vi "Set Log Trigger Default Value.vi"(8 "error in":errorcluster, 10 "log trigger default value":bool, 11 "log file in":T1 format="%.0x") -> (0 "error out":errorcluster, 3 "log file out":T1 format="%.0x")   [LabVIEW 2027, in "Embedded Data Logger Scripting.lvlib"]
uses:
  Embedded Data Logger Scripting.lvlib
  <vilib>/NI VeriStand/Custom Device API/Custom Device Item Ref.ctl
  Shared/Constants.vi
  <vilib>/NI VeriStand/Custom Device Tools/Custom Device Utility Library/NI VeriStand - Search for Item by GUID.vi
  <vilib>/NI VeriStand/Custom Device Tools/Custom Device Utility Library/Custom Device Utility Library.lvlib
  Shared/Embedded Data Logger Shared.lvlib
  <vilib>/NI VeriStand/Custom Device API/Custom Device API.lvlib
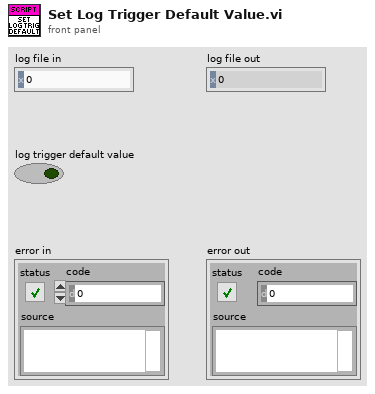
[diagram p1: front panel]
types:
  T1 = typedef "Custom Device API.lvlib/Custom Device Item Ref.ctl" = u64
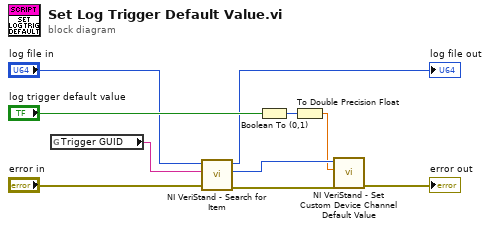
[diagram p0: block diagram]
diagram:
  n1 = global read "Constants.vi" "Trigger GUID"() -> (w9:string)
  n2 = call-poly <vilib>:"NI VeriStand - Search for Item.vi"("error in"="error in", "Item GUID"=w9, "Section Ref in"="log file in") -> ("error out"=w7:errorcluster, "Item Ref"=w6:T1, "Section Ref out"=→"log file out":T1)  [unwired: 5 in, 1 out]
  n3 = Boolean To (0,1)(Boolean="log trigger default value") -> (0, 1=w4:i16)
  n4 = To Double Precision Float(number=w4) -> (double precision float=w3:dbl)
  n5 = call <vilib>:"NI VeriStand - Set Custom Device Channel Default Value.vi"("error in (no error)"=w7, "Default Value"=w3, "Channel Ref in"=w6) -> ("error out"=→"error out":errorcluster)  [unwired: 7 in, 1 out]
